vi "getLiveXT.vi"() -> (0 "T-Axis Offset":dbl, 1 "X-Axis Offset":dbl, 2 "transposed array":dbl[][](array[numeric]), 3 "LiveImageXT_ArrayData":dbl[](array[numeric]))   [LabVIEW 2018]
uses:
  <userlib>/caLab/Private/Get_PV.vi
panel:
  out "Intensity Graph":dbl[][](graph)
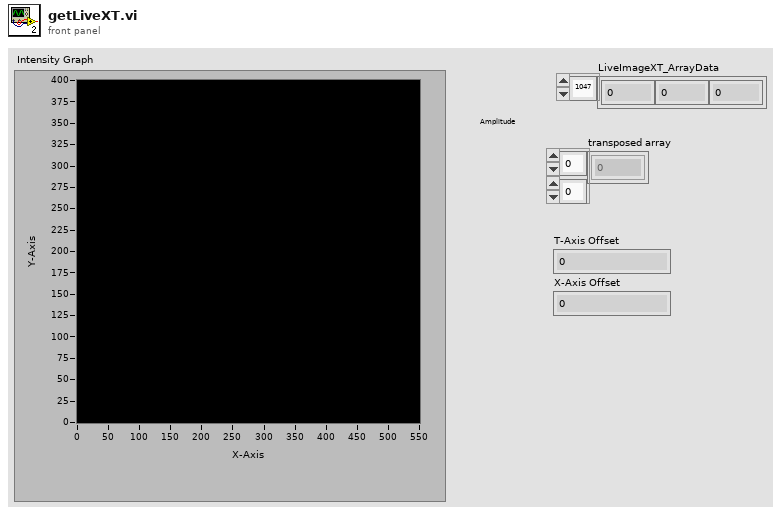
[diagram p1: front panel]
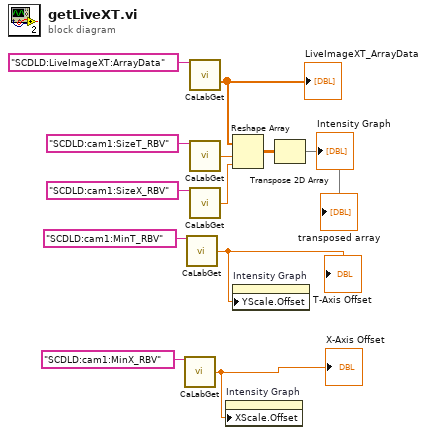
[diagram p0: block diagram]
diagram:
  n1 = call-poly <userlib>:"CaLabGet.vi"("PV Name"="SCDLD:cam1:MinX_RBV") -> ("1rst Value (number)"=w1:dbl)  [unwired: 8 in, 6 out]
  "X-Axis Offset" <- w1
  n2 = call-poly <userlib>:"CaLabGet.vi"("PV Name"="SCDLD:cam1:MinT_RBV") -> ("1rst Value (number)"=w2:dbl)  [unwired: 8 in, 6 out]
  "T-Axis Offset" <- w2
  n3 = call-poly <userlib>:"CaLabGet.vi"("PV Name"="SCDLD:LiveImageXT:ArrayData") -> ("Value Array (number)"=w10:dbl[])  [unwired: 8 in, 6 out]
  "LiveImageXT_ArrayData" <- w10
  n4 = call-poly <userlib>:"CaLabGet.vi"("PV Name"="SCDLD:cam1:SizeT_RBV") -> ("1rst Value (number)"=w4:dbl)  [unwired: 8 in, 6 out]
  n5 = call-poly <userlib>:"CaLabGet.vi"("PV Name"="SCDLD:cam1:SizeX_RBV") -> ("1rst Value (number)"=w3:dbl)  [unwired: 8 in, 6 out]
  n6 = property on="Intensity Graph" class="IntGraph (strict)"("XScale.Offset"=w1) -> ()  [unwired: 2 in, 2 out]
  n7 = Reshape Array(w10, w4, w3) -> (w11:dbl[][])
  n8 = property on="Intensity Graph" class="IntGraph (strict)"("YScale.Offset"=w2) -> ()  [unwired: 2 in, 2 out]
  n9 = Transpose 2D Array(2D array=w11) -> (transposed array=→"Intensity Graph" →"transposed array":dbl[][])
